vi "CreatePublicEvents.vi"(8 "error in (no error)":errorcluster, 11 "MeasuringDevice":refnum<class "MeasuringDevice.lvclass">) -> (0 "error out":errorcluster, 3 "MeasuringDevice out":refnum<class "MeasuringDevice.lvclass">)   [LabVIEW 2017, in "MeasuringDevice.lvclass"]
doc: "---------------------------------------------------------------\nJKI State Machine Objects™\nhttp://jki.net/state-machine-objects/\nCopyright (C) 2005-2015, JKI <info@jki.net>\nALL RIGHTS RESERVEDJKI State Machine Objects (SMO) 1.0.0.5\nJKI - JKI\nCopyright (c) 2016, JKI"
uses:
  MeasuringDevice.lvclass
  MeasuringDevice.lvclass/MeasuringDevice.ctl
  Typedefs/PublicEvents--MeasuringDevice.MeasurementCompleted.ctl
  <vilib>/JKI/JKI SMO/SMO/SMO.lvclass
panel:
  # "For instructions on how to use the JKI State Machine Objects, examples and video tutorials, visit:\nhttp://jki.net/state-machine-objects/\n\nJKI State Machine Objects™\nhttp://jki.net/state-machine-objects/\nCopyright (C) 2005-2015, JKI <info@jki.net>\nALL RIGHTS RESERVED"
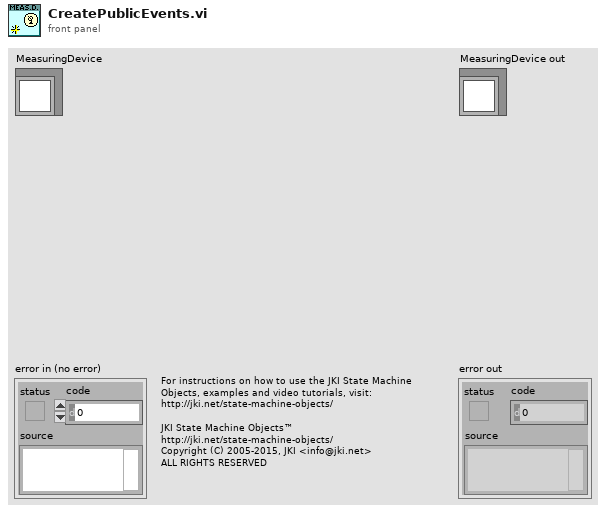
[diagram p1: front panel]
types:
  T1 = typedef "MeasuringDevice.lvclass/PrivateData--Ref.ctl" = refnum<data-value>
  T2 = typedef "MeasuringDevice.lvclass/PublicEvents--MeasuringDevice.MeasurementCompleted.ctl" = i32
  T3 = typedef "MeasuringDevice.lvclass/PrivateData--Cluster.ctl" = cluster{"Public Events":T4, "Private Events":T5, "Dependencies":T6}
  T4 = typedef "MeasuringDevice.lvclass/PublicEvents--Cluster.ctl" = cluster{"MeasurementCompleted":refnum<user-event>}
  T5 = typedef "MeasuringDevice.lvclass/PrivateEvents--Cluster.ctl" = cluster{"MakeMeasurement":refnum<user-event>}
  T6 = typedef "MeasuringDevice.lvclass/Dependencies--Cluster.ctl" = cluster{"MeasurementBuffer":refnum<class "CircularBuffer.lvclass">}
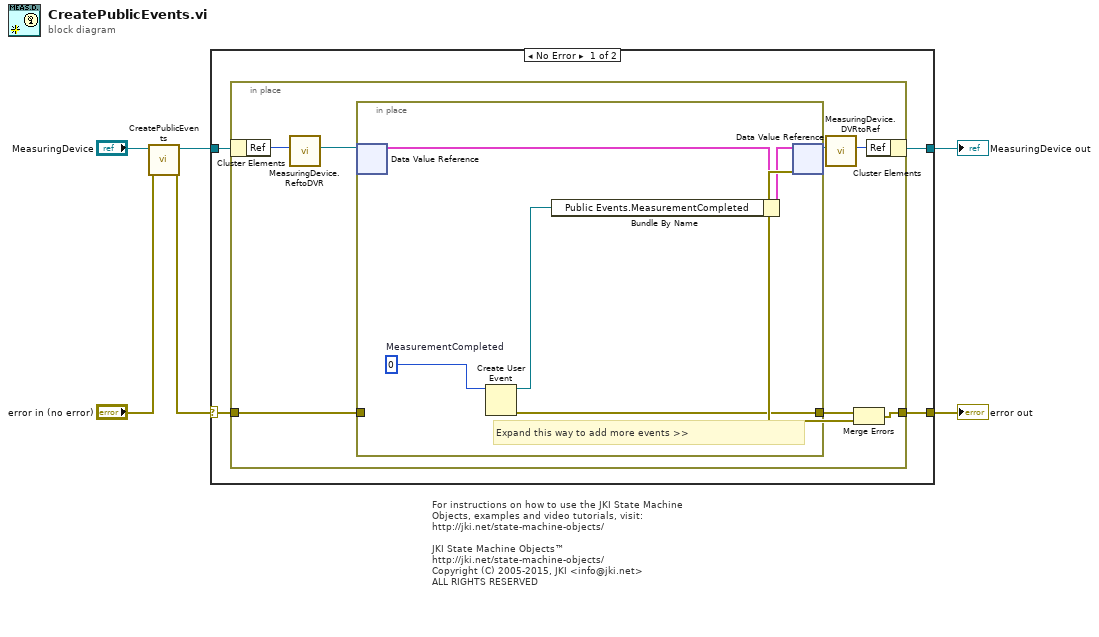
[diagram p0: block diagram]
diagram:
  # "For instructions on how to use the JKI State Machine Objects, examples and video tutorials, visit:\nhttp://jki.net/state-machine-objects/\n\nJKI State Machine Objects™\nhttp://jki.net/state-machine-objects/\nCopyright (C) 2005-2015, JKI <info@jki.net>\nALL RIGHTS RESERVED"
  n1 = call-parent "CreatePublicEvents.vi"("error in (no error)"="error in (no error)", "SMO"="MeasuringDevice") -> ("error out"=w1:errorcluster, "SMO out"=w3:refnum<class "MeasuringDevice.lvclass">)  [unwired: 8 in]
  n2 = case shown="No Error" w1 {
    selector: w1 -> [w8 w25]
    tunnel: [w7 w25] -> w5
    tunnel: [w9 w24] -> w6
    tunnel: w3 -> [w10 w24]
    frame No Error {
      n3 = in-place {
        in-place-border: w8 -> [w18]
        in-place-border: [w15] -> w7
        n4 = in-place-cluster #1(w10) -> ("Ref"=w14:u32)
        n5 = call "MeasuringDevice.ReftoDVR.vi"("Ref"=w14) -> ("Ref"=w13:T1)  [unwired: 10 in]
        n6 = in-place {
          in-place-border: w18 -> [_]
          in-place-border: [w21] -> w17
          w20 = T2 0  # MeasurementCompleted
          # "Expand this way to add more events >>"
          n7 = in-place-dvr #2(w13) -> (w22:T3)  [unwired: 1 out]
          n8 = Create User Event(user event datatype=w20) -> (user event=w19:refnum<user-event>, error out=w21:errorcluster)  [unwired: 1 in]
          n9 = Bundle By Name(cluster=w22, "Public Events.MeasurementCompleted"=w19) -> (w23:T3)
          n10 = in-place-dvr #2(w23) -> (w12:T1, w16:errorcluster)
        }
        n11 = call "MeasuringDevice.DVRtoRef.vi"("Ref"=w12) -> ("Ref"=w11:u32)  [unwired: 10 in]
        n12 = Merge Errors(w17, w16) -> (w15:errorcluster)
        n13 = in-place-cluster #1("Ref"=w11) -> (w9:refnum<class "MeasuringDevice.lvclass">)
      }
    }
    frame Error {
    }
  }
  "error out" <- w5
  "MeasuringDevice out" <- w6
